vi "untriggered_stimulus_functional_global.vi"() -> ()   [LabVIEW 2019]
uses:
  BufferStimulusFunctionalGlobalOperations.ctl
  ParametersGlobal.vi
  StimulusObject.lvclass
panel:
  out "UntriggeredStimulusOut":sgl[][](array[numeric])
  out "error out":errorcluster
  in  "error in (no error)":errorcluster
  in  "Operation":T1
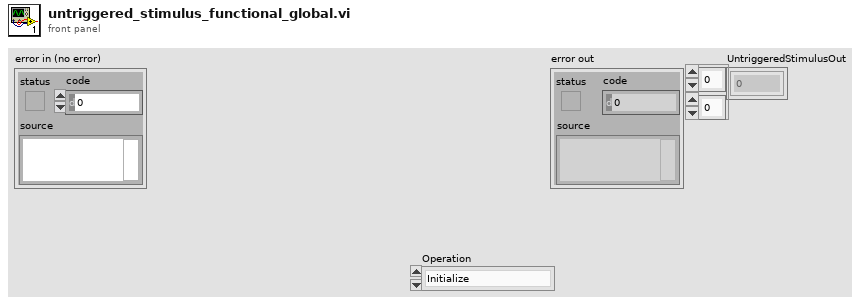
[diagram p1: front panel]
types:
  T1 = typedef "BufferStimulusFunctionalGlobalOperations.ctl" = enum16{"Initialize", "Buffer", "GetOne", "GetTwo"}
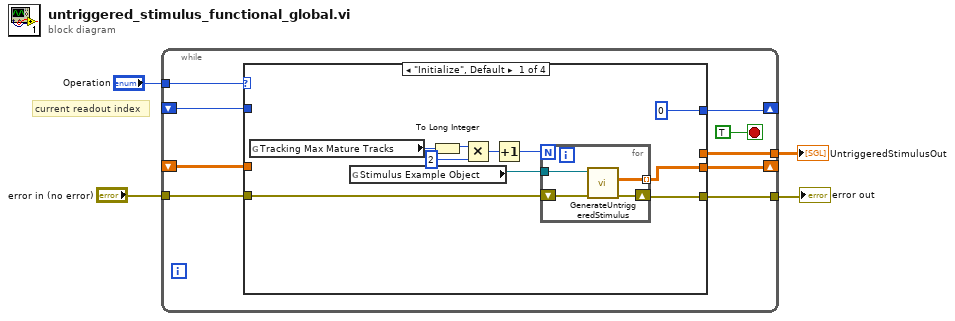
[diagram p0: block diagram]
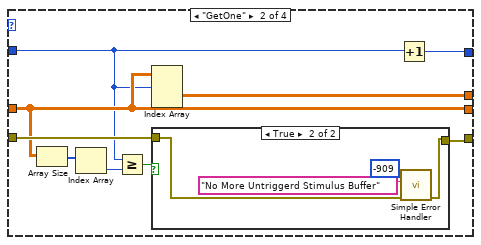
[diagram p2: hidden frame]
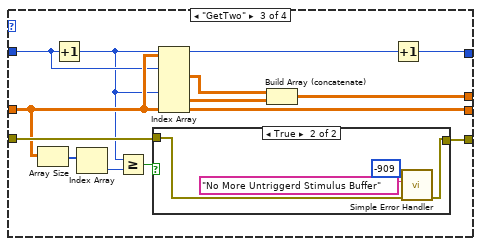
[diagram p4: hidden frame]
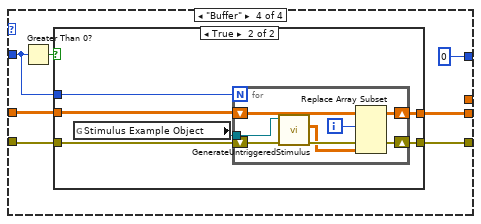
[diagram p6: hidden frame]
diagram:
  # "current readout index"
  n1 = while {
    tunnel: "Operation" -> [w12]
    tunnel: "error in (no error)" -> [w11]
    tunnel: [w10] -> w2
    shift-right: [w9] -> _
    shift-left: _ -> [w8]
    shift-right: [w7] -> _
    shift-left: _ -> [w6]
    tunnel: [w5] -> w1
    stop <- TRUE stop-if-true
    n2 = case shown="\"Initialize\", Default" w12 {
      tunnel: w11 -> [w23 w35 w48 w64]
      tunnel: [w22 w34 w49 w63] -> w10
      tunnel: [w14 w30 w47 w60] -> w9
      tunnel: w8 -> [_ w30 w47 w61]
      tunnel: [0 ("x-1") w31 w53 0 ("x-1")] -> w7
      tunnel: w6 -> [_ w29 w46 w59]
      tunnel: [_ w28 w42 _] -> w5
      frame "Initialize", Default {
        n3 = global read "ParametersGlobal.vi" "Tracking Max Mature Tracks"() -> (w20:i16)
        n4 = global read "ParametersGlobal.vi" "Stimulus Example Object"() -> (w21:refnum<class "StimulusObject.lvclass">)
        n5 = To Long Integer(number=w20) -> (32bit integer=w17:i32)
        n6 = Multiply(x=w17, y=2) -> (x*y=w15:i32)
        n7 = Increment(x=w15) -> (x+1=w18:i32)
        n8 = for {
          N: w18 -> [_]
          tunnel: w21 -> [w25]
          shift-right: [w26] -> w22
          shift-left: w23 -> [w27]
          tunnel: [w24] -> w14 mode=indexing
          n9 = call-dynamic "GenerateUntriggeredStimulus.vi"("error in (no error)"=w27, "StimulusObject in"=w25) -> ("error out"=w26:errorcluster, "UntriggeredStimulusOut"=w24:sgl[][])  [unwired: 7 in, 1 out]
        }
      }
      frame "GetOne" {
        n10 = Array Size(array=w30) -> (size(s)=w33:i32[])
        n11 = Index Array(array=w33) -> (element=w32:i32)  [unwired: 1 in]
        n12 = Greater Or Equal?(x=w29, y=w32) -> (x >= y?=w36:bool)
        n13 = Index Array(array=w30, index (dim 0)=w29) -> (element=w28:sgl[][])  [unwired: 2 in]
        n14 = case shown="True" w36 {
          tunnel: w35 -> [w37 w39]
          tunnel: [w37 w38] -> w34
          frame False {
          }
          frame True {
            n15 = call <vilib>:"Simple Error Handler.vi"("error code (no error:0)"=-909, "error source (\" \")"="No More Untriggerd Stimulus Buffer" ("error source (\" \")"), "error in (no error)"=w39) -> ("error out"=w38:errorcluster)  [unwired: 2 in, 4 out]
          }
        }
        n16 = Increment(x=w29) -> (x+1=w31:i32)
      }
      frame "GetTwo" {
        n17 = Array Size(array=w47) -> (size(s)=w51:i32[])
        n18 = Increment(x=w46) -> (x+1=w45:i32)
        n19 = Index Array(array=w51) -> (element=w50:i32)  [unwired: 1 in]
        n20 = Greater Or Equal?(x=w45, y=w50) -> (x >= y?=w52:bool)
        n21 = case shown="True" w52 {
          tunnel: w48 -> [w54 w56]
          tunnel: [w54 w55] -> w49
          frame False {
          }
          frame True {
            n22 = call <vilib>:"Simple Error Handler.vi"("error code (no error:0)"=-909, "error source (\" \")"="No More Untriggerd Stimulus Buffer" ("error source (\" \")"), "error in (no error)"=w56) -> ("error out"=w55:errorcluster)  [unwired: 2 in, 4 out]
          }
        }
        n23 = Index Array(array=w47, index (dim 0) #1=w46, index (dim 0) #2=w45) -> (element #1=w44:sgl[][], element #2=w43:sgl[][])  [unwired: 4 in]
        n24 = Build Array (concatenate)(w44, w43) -> (w42:sgl[][])
        n25 = Increment(x=w45) -> (x+1=w53:i32)
      }
      frame "Buffer" {
        n26 = Greater Than 0?(x=w59) -> (x > 0?=w62:bool)
        n27 = case shown="True" w62 {
          tunnel: w64 -> [w66 w73]
          tunnel: [w66 w72] -> w63
          tunnel: w61 -> [w67 w70]
          tunnel: [w67 w69] -> w60
          tunnel: w59 -> [_ w68]
          frame False {
          }
          frame True {
            n28 = global read "ParametersGlobal.vi" "Stimulus Example Object"() -> (w71:refnum<class "StimulusObject.lvclass">)
            n29 = for {
              N: w68 -> [_]
              tunnel: w71 -> [w78]
              shift-right: [w79] -> w72
              shift-left: w73 -> [w80]
              shift-right: [w74] -> w69
              shift-left: w70 -> [w77]
              i -> [w76]
              n30 = call-dynamic "GenerateUntriggeredStimulus.vi"("error in (no error)"=w80, "StimulusObject in"=w78) -> ("error out"=w79:errorcluster, "UntriggeredStimulusOut"=w75:sgl[][])  [unwired: 7 in, 1 out]
              n31 = Replace Array Subset(array=w77, new element=w75, index (dim 0)=w76) -> (w74:sgl[][][])  [unwired: 2 in]
            }
          }
        }
      }
    }
  }
  "error out" <- w2
  "UntriggeredStimulusOut" <- w1
